vi "GDC Befehl empfangen.vi"(8 "error in (no error)":errorcluster caption="Fehler (Eingang, kein Fehler)", 11 "VISA-Ressourcenname":refnum<visa-resource-name>) -> (0 "error out":errorcluster caption="Fehler (Ausgang)", 1 "Daten":string, 2 "Befehl":string, 3 "VISA-Ressourcenname (Ausgang)":refnum<visa-resource-name>)   [LabVIEW 2020, in "Linearisierung v2.lvlib" / "Gasteiler.lvlib" / "Horiba GDC.lvlib"]
uses:
  Horiba GDC.lvlib
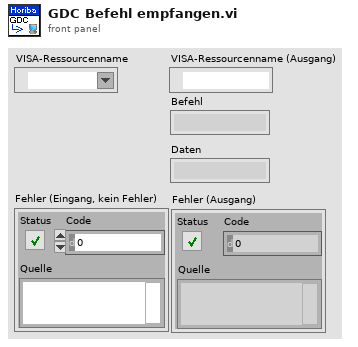
[diagram p1: front panel]
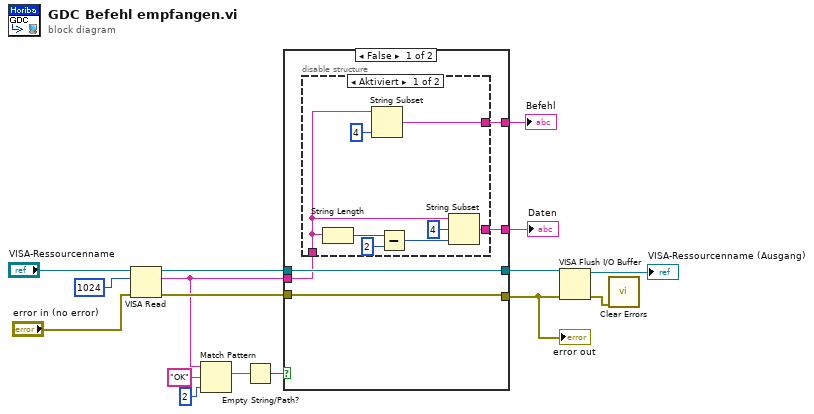
[diagram p0: block diagram]
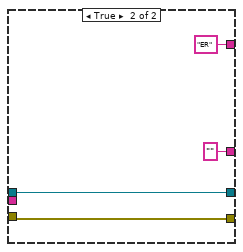
[diagram p3: hidden frame]
diagram:
  n1 = VISA Read(VISA resource name="VISA-Ressourcenname", byte count=u32 1024 ("Byte-Anzahl"), error in (no error)="error in (no error)") -> (VISA resource name out=w3:refnum<visa-resource-name>, read buffer=w2:string, error out=w8:errorcluster)  [unwired: 1 out]
  n2 = Match Pattern(string=w2, regular expression="OK" ("Regulärer Ausdruck"), offset (0)=2 ("Offset (0)")) -> (match substring=w12:string)  [unwired: 3 out]
  n3 = Empty String/Path?(string/path=w12) -> (empty?=w11:bool)
  n4 = case shown="False" w11 {
    tunnel: w2 -> [w18 _]
    tunnel: w3 -> [w21 w34]
    tunnel: [w21 w34] -> w10
    tunnel: w8 -> [w20 w33]
    tunnel: [w20 w33] -> w1
    tunnel: [w19 "" ("read buffer")] -> w5
    tunnel: [w17 "ER" ("read buffer")] -> w4
    frame False {
      n5 = disable-structure shown="Aktiviert" {
        disable-tunnel: [w28 w30] -> w19
        disable-tunnel: w18 -> [w23 w30]
        disable-tunnel: [w22 _] -> w17
        frame Enabled {
          n6 = String Length(string=w23) -> (length=w27:i32)
          n7 = String Subset(string=w23, length (rest)=4 ("Länge (Rest)")) -> (substring=w22:string)  [unwired: 1 in]
          n8 = Subtract(x=w27, y=2) -> (x-y=w25:i32)
          n9 = String Subset(string=w23, offset (0)=4 ("Offset (0)"), length (rest)=w25) -> (substring=w28:string)
        }
        frame Disabled {
        }
      }
    }
    frame True {
    }
  }
  "error out" <- w1
  "Daten" <- w5
  "Befehl" <- w4
  n10 = VISA Flush I/O Buffer(VISA resource name=w10, error in (no error)=w1) -> (VISA resource name out=→"VISA-Ressourcenname (Ausgang)":refnum<visa-resource-name>, error out=w7:errorcluster)  [unwired: 1 in]
  n11 = call <vilib>:"Clear Errors.vi"("error in (no error)"=w7) -> ()  [unwired: 5 in, 2 out]
